vi "Endpoints.vi"(6 "Template in":string, 7 "Action":T1, 8 "VI Refnum in":refnum<vi>, 9 "Content-Type in":string, 10 "Content in":string, 11 "Endpoint":string) -> (0 "VI Refnum out":refnum<vi>, 1 "Content-Type out":string, 2 "Content out":string, 3 "Found?":bool, 4 "Template out":string, 5 "Endpoints":string[](array[string]))   [LabVIEW 2021, in "HttpServer.lvlib"]
uses:
  HttpServer.lvlib
  TypeDefs/Action.ctl
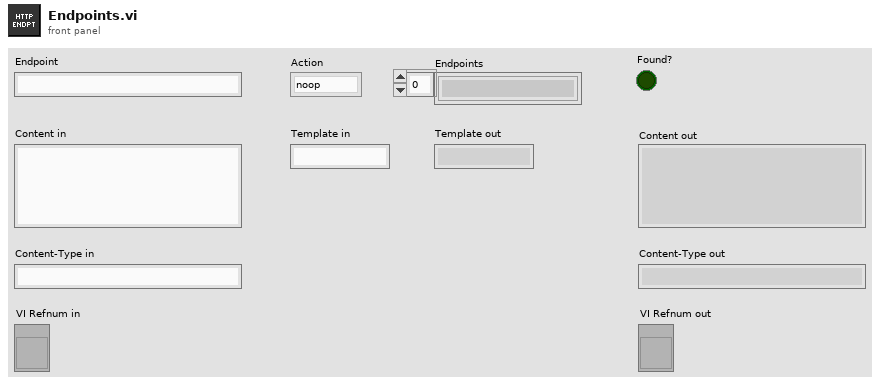
[diagram p1: front panel]
types:
  T1 = typedef "HttpServer.lvlib/Action.ctl" = enum8{"noop", "add", "get", "set", "remove"}
  T2 = map{string, cluster{"Content":string, "Content-Type":string, "VI Refnum":refnum<vi>, "Template":string}}
  T3 = cluster{"Content in":string, "Content-Type in":string, "VI Refnum in":refnum<vi>, "Template in":string}
  T4 = cluster{"Content":string, "Content-Type":string, "VI Refnum":refnum<vi>, "Template":string}
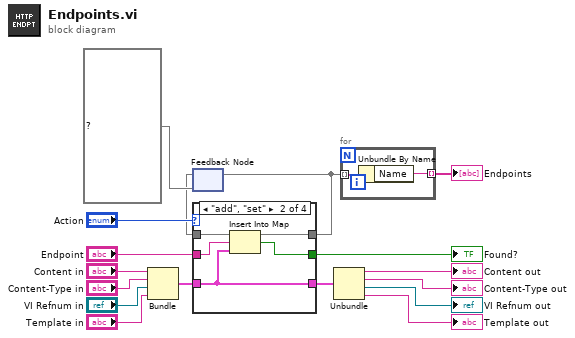
[diagram p0: block diagram]
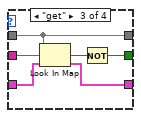
[diagram p3: hidden frame]
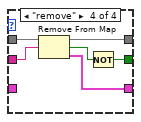
[diagram p4: hidden frame]
diagram:
  n1 = Bundle("Content in"="Content in", "Content-Type in"="Content-Type in", "VI Refnum in"="VI Refnum in", "Template in"="Template in") -> (w8:T3)  [unwired: 1 in]
  n2 = feedback #1(T2 {} ("Templates")) -> (w15:T2)
  n3 = case shown="\"add\", \"set\"" "Action" {
    tunnel: w15 -> [w18 w23 w29 w35]
    tunnel: [w18 w22 w29 w34] -> w12
    tunnel: "Endpoint" -> [_ w21 w28 w33]
    tunnel: w8 -> [_ w19 w27 _]
    tunnel: [_ w19 w26 w32] -> w10
    tunnel: [_ w20 w24 w30] -> w9
    frame "noop" {
    }
    frame "add", "set" {
      n4 = Insert Into Map(map in=w23, key=w21, value=w19) -> (map out=w22:T2, key already included?=w20:bool)  [unwired: 1 out]
    }
    frame "get" {
      n5 = Look In Map(map=w29, key=w28, default value=w27) -> (key not found?=w25:bool, value=w26:T3)
      n6 = Not(x=w25) -> (.not. x?=w24:bool)
    }
    frame "remove" {
      n7 = Remove From Map(10:w33, 11:w35) -> (1:w32:T4, 2:w31:bool, 3:w34:T2)
      n8 = Not(x=w31) -> (.not. x?=w30:bool)
    }
  }
  "Found?" <- w9
  n9 = feedback-in #1(w12) -> ()
  n10 = Unbundle(w10) -> ("Content"=→"Content out":string, "Content-Type"=→"Content-Type out":string, "VI Refnum"=→"VI Refnum out":refnum<vi>, "Template"=→"Template out":string)
  n11 = for {
    tunnel: w12 -> [w37] mode=indexing
    tunnel: [w36] -> w11 mode=indexing
    n12 = Unbundle By Name(w37) -> ("Name"=w36:string)
  }
  "Endpoints" <- w11
